vi "Main.vi"() -> ()   [LabVIEW 2018]
panel:
  in  "选项卡控件":enum32{"主页", "设置"}(tab)
  in  "确定按钮":bool
  in  "路径":path=path "C:/Users/Twsa/Documents/Graduction-Project/send_test.txt"
  in  "端口号":refnum<visa-resource-name>="COM4"
  in  "每次发送大小":i32=10240
  in  "波特率":u32=9600
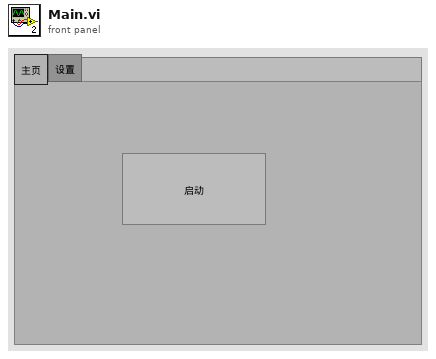
[diagram p1: front panel]
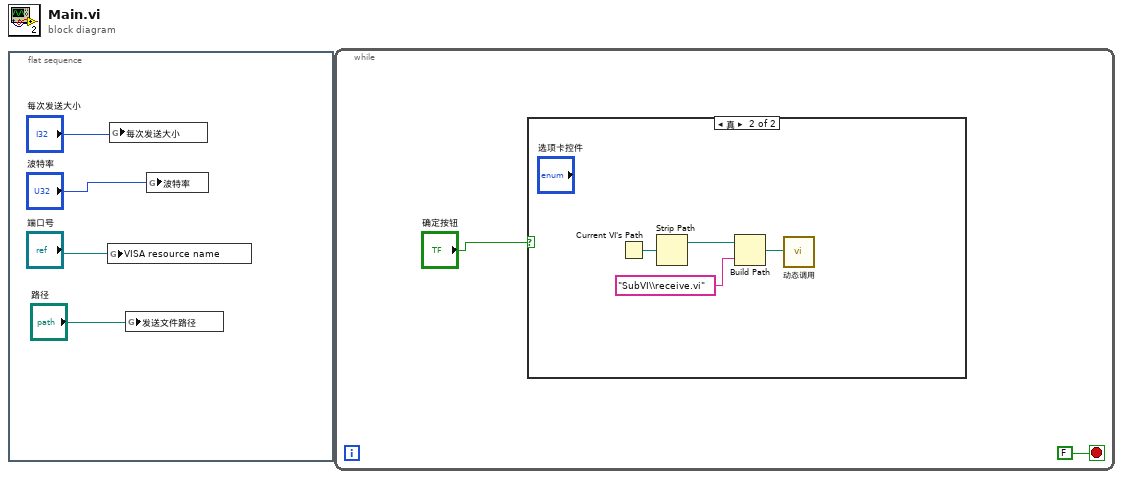
[diagram p0: block diagram]
diagram:
  n1 = flat-sequence {
    frame #0 {
      n2 = global write "全局变量.vi" "VISA resource name"("端口号") -> ()
      n3 = global write "全局变量.vi" "每次发送大小"("每次发送大小") -> ()
      n4 = global write "全局变量.vi" "发送文件路径"("路径") -> ()
      n5 = global write "全局变量.vi" "波特率"("波特率") -> ()
    }
  }
  n6 = while {
    stop <- FALSE stop-if-true
    n7 = case shown="真" "确定按钮" {
      frame False {
      }
      frame True {
        n8 = Current VI's Path() -> (path=w8:path)
        n9 = Strip Path(path=w8) -> (stripped path=w9:path)  [unwired: 1 out]
        n10 = Build Path(base path=w9, name or relative path="SubVI\\receive.vi" ("名称或相对路径")) -> (appended path=w10:path)
        n11 = call "动态调用.vi"("VI路径"=w10) -> ()  [unwired: 11 in]
      }
    }
  }
